vi "Pfeiffer_Offset_Display.vi"(5 "Port":i32(ring) items=["COM 1", "COM 2", "COM 3", "COM 4", "COM 5", "COM 6", "COM 7", "COM 8", "COM 9", "COM 10", "COM 11", "COM 12"], 6 "Error In":bool, 7 "W/R":bool, 8 "Sensor 2 Set":dbl format="%.3e", 9 "Sensor 1 Set":dbl format="%.3e") -> (0 "Sensor2 Get":dbl format="%.3e", 1 "Sensor 1 Get":dbl format="%.3e", 4 "Error Out":bool)   [LabVIEW 2010]
doc: "VI runs with Single / Dual Gauge (TPG 252 / 261 / 262)"
panel:
  # "mbar"
  # "mbar"
  # "mbar"
  # "mbar"
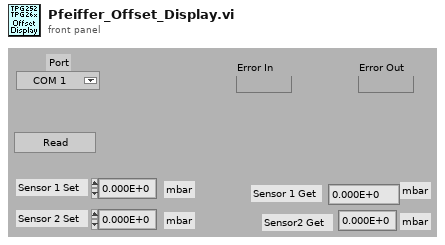
[diagram p1: front panel]
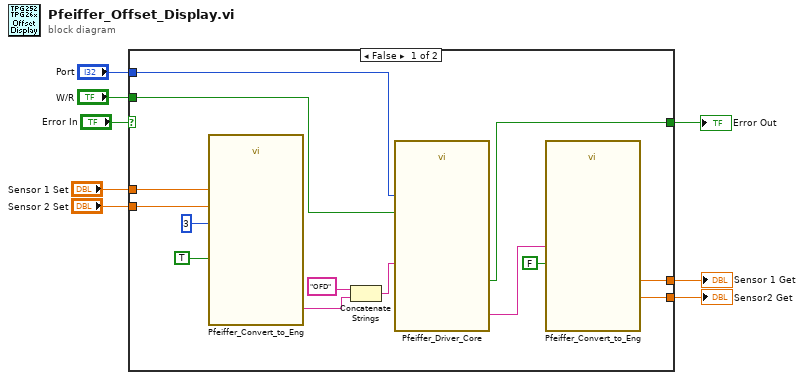
[diagram p0: block diagram]
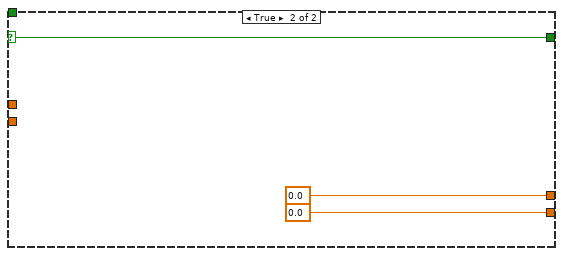
[diagram p2: hidden frame]
diagram:
  n1 = case shown="False" "Error In" {
    selector: "Error In" -> [_ w25]
    tunnel: "Port" -> [w22 _]
    tunnel: "W/R" -> [w21 _]
    tunnel: [w14 w25] -> w5
    tunnel: "Sensor 1 Set" -> [w13 _]
    tunnel: "Sensor 2 Set" -> [w12 _]
    tunnel: [w11 0.0 ("Eng1 out")] -> w2
    tunnel: [w10 0.0 ("Eng2 out")] -> w1
    frame False {
      n2 = call "Pfeiffer_Convert_to_Eng.vi"("W/R [W: Int in; Str out ]"=TRUE, "Kommastellen"=u8 3, "Eng2 in"=w12, "Eng1 in"=w13) -> ("String out"=w18:string)  [unwired: 1 in, 6 out]
      n3 = Concatenate Strings("OFD" ("Command"), w18) -> (w17:string)
      n4 = call "Pfeiffer_Driver_Core.vi"("Command"=w17, "Write/Read"=w21, "Port"=w22) -> ("String Out"=w15:string, "Error"=w14:bool)  [unwired: 2 in, 9 out]
      n5 = call "Pfeiffer_Convert_to_Eng.vi"("W/R [W: Int in; Str out ]"=FALSE, "String in"=w15) -> ("Eng2 out"=w10:dbl, "Eng1 out"=w11:dbl)  [unwired: 3 in, 5 out]
    }
    frame True {
    }
  }
  "Error Out" <- w5
  "Sensor2 Get" <- w1
  "Sensor 1 Get" <- w2
